vi "EdF.vi"() -> ()   [LabVIEW 2016]
doc: "EdF Test Program - application for testing RadICS platform logic for EdF Project"
uses:
  TypeDef/State.ctl
  TypeDef/Cluster.ctl
  <vilib>/DAQmx/write.llb/DAQmx Write (Digital 1D Bool 1Chan 1Samp).vi
  <vilib>/DAQmx/write.llb/DAQmx Write (Analog 1D DBL NChan 1Samp).vi
  <vilib>/DAQmx/read.llb/DAQmx Read (Digital 1D Bool 1Chan 1Samp).vi
  <vilib>/DAQmx/read.llb/DAQmx Read (Analog 1D DBL NChan 1Samp).vi
  <vilib>/DAQmx/create/channels.llb/DAQmx Create Channel (AO-Voltage-Basic).vi
  <vilib>/DAQmx/create/channels.llb/DAQmx Create Channel (AI-Voltage-Basic).vi
  <vilib>/DAQmx/create/channels.llb/DAQmx Create Channel (DO-Digital Output).vi
  <vilib>/DAQmx/create/channels.llb/DAQmx Create Channel (DI-Digital Input).vi
  <vilib>/DAQmx/miscellaneous.llb/DAQmx Fill In Error Info.vi
  <resource>/objmgr/daqmx.rc
panel:
  in  "PrntScr":bool
  in  "AddTab":enum32{"Page 1"}(tab)
  in  "PID":bool
  in  "Run":bool
  in  "Clear":bool
  out "Graph":dbl[][](graph)
  in  "stop":bool
  in  "Tab":T1(tab)
  in  "AO":tag="6704_S2/ao0:1"
  in  "AI":tag="6224_S4/ai16:21"
  in  "DO":tag="6513_S5/port0/line0:7, 6513_S5/port1/line0:7, 6513_S5/port2/line0"
  in  "DI":tag="6511_S6/port0/line0:7, 6511_S6/port1/line0:3"
  in  "D_out":bool[](array[boolean]) caption="Digital output"
  in  "V_out":dbl[](array[knob]) caption="Analog output,  V" min=0.0 max=5.0 step=1.0 scale=0.0..5.0 scale format="%#.3g"
  in  "AO Names":string[](array[string])=["SRI_2101_MT", "SRI_2203_MT"]
  out "V_in":dbl[](array[numeric]) caption="Analog input, V" format="%.3g"
  in  "AI Names":string[](array[string])=["SRI_01_02_VA_HMI", "SRI_2103_VA_HMI", "SRI_2203MT_HMI", "SRI_2101_VA", "SRI_2102_VA", "SRI_2103_VA"]
  in  "Delay, ms":i32=200
  in  "buf_size":i32=1000 caption="Graph buffer size"
  in  "PID buff":i32=100 caption="PID buffer size"
  in  "DO Names":string[](array[string])=["SRI_2101_RGp_HMI", "SRI_2101_RGm_HMI", "SRI_2101_MA_HMI", "SRI_2150_VN4", "SRI_2160_VN4", "SRI_1201_SN1", "SRI_1202_SN1", "SRI_1203_SN1", "SRI_1201_SN2", "SRI_1202_SN2", "SRI_1203_SN2", "SRI_1101_EE", "SRI_1101_DE", "SRI_1102_EE", "SRI_1102_DE", "SRI_1103_EE", "SRI_1103_DE"]
  out "D_in":bool[](array[boolean]) caption="Digital input"
  in  "DI Names":string[](array[string])=["SRI_2101_AA_HMI", "SRI_2102_AA_HMI", "SRI_1201_AA_HMI", "SRI_1202_AA_HMI", "SRI_1203_AA_HMI", "SER_1201_VA", "SRI_1101_OF", "SRI_1102_OF", "SRI_1103_OF", "SRI_1101_ON", "SRI_1102_ON", "SRI_1103_ON"]
  in  "2203MT":dbl caption="SRI 2203 MT ( C)" min=0.0 max=40.0 step=1.0
  out "03MT":dbl caption="SRI 2203 MT ( C)" format="%.3g"
  out "2103VA":dbl caption="SRI 2103 VA (%)" format="%.3g"
  out "0102VA":dbl caption="SRI 2101/02 VA (%)" format="%.3g"
  in  "2101MT":dbl caption="SRI 2101 MT ( C)" min=0.0 max=40.0 step=1.0
  in  "01RGp":bool caption="SRI 2101 RG+"
  in  "01RGm":bool caption="SRI 2101 RG-"
  in  "01MA":bool caption="SRI 2101 MA"
  in  "50VN4":bool caption="SRI 2150 VN4 (DI)"
  in  "60VN4":bool caption="SRI 2160 VN4 (DI)"
  out "03VA":dbl caption="SRI 2103 VA (%)" format="%.3g"
  out "02AA 2":bool caption="SRI 2102 AA (HMI)"
  out "01AA 2":bool caption="SRI 2101 AA (HMI)"
  out "01VA 2":dbl caption="SRI 2101 VA (%)" format="%.3g"
  out "02VA":dbl caption="SRI 2102 VA (%)" format="%.3g"
  out "03OF":bool caption="SRI 1103 OF (DO)"
  out "01OF":bool caption="SRI 1101 OF (DO)"
  out "02OF":bool caption="SRI 1102 OF (DO)"
  in  "03DE":bool caption="SRI 1103 DE (DI)"
  in  "03EE":bool caption="SRI 1103 EE (DI)"
  in  "02DE":bool caption="SRI 1102 DE (DI)"
  in  "02EE":bool caption="SRI 1102 EE (DI)"
  in  "01DE":bool caption="SRI 1101 DE (DI)"
  out "03ON":bool caption="SRI 1103 ON (DO)"
  out "01ON":bool caption="SRI 1101 ON (DO)"
  out "02ON":bool caption="SRI 1102 ON (DO)"
  in  "01EE":bool caption="SRI 1101 EE (DI)"
  out "03AA":bool caption="SRI 1203 AA"
  out "01VA":bool caption="SER 1201 VA"
  out "02AA":bool caption="SRI 1202 AA"
  in  "01SN1":bool caption="SRI 1201 SN1 (DI)"
  in  "02SN1":bool caption="SRI 1202 SN1 (DI)"
  in  "03SN1":bool caption="SRI 1203 SN1 (DI)"
  in  "01SN2":bool caption="SRI 1201 SN2 (DI)"
  in  "03SN2":bool caption="SRI 1203 SN2 (DI)"
  in  "02SN2":bool caption="SRI 1202 SN2 (DI)"
  out "01AA":bool caption="SRI 1201 AA"
  # "o"
  # "Program Settings"
  # "Closed Loop Control Operation"
  # "0,6648"
  # "0,33"
  # "o"
  # "o"
  # "S0"
  # "D0"
  # "Y"
  # "0,0"
  # "COM"
  # "D1"
  # "0,2"
  # "o"
  # "D0"
  # "Y"
  # "COM"
  # "D1"
  # "S0"
  # "in_1"
  # "out"
  # "OR"
  # "in_2"
  # "op1"
  # "o_result"
  # "SUB"
  # "op2"
  # "op1"
  # "o_result"
  # "MUL"
  # "op2"
  # "op1"
  # "o_result"
  # "MUL"
  # "op2"
  # "o"
  # "17 C"
  # "in_a"
  # "out a<b"
  # "CMP"
  # "in_b"
  # "in_a"
  # "out a>b"
  # "CMP"
  # "in_b"
  # "o"
  # "30 C"
  # "o"
  # "16 C"
  # "op1"
  # "o_result"
  # "SUB"
  # "op2"
  # "i_plus"
  # "o_x_act"
  # "RG"
  # "i_minus"
  # "i_man"
  # "i_x_auto"
  # "o_auto"
  # "i_err"
  # "o_ctrl_val"
  # "PID"
  # "i_prev"
  # "i_auto"
  # "Normal/backup pump operation"
  # "PO3"
  # "PO1"
  # "PO1"
  # "PO2"
  # "PO2"
  # "PO3"
  # "Niv_BAS_01BA"
  # "tctc_vibr"
  # "in"
  # "out"
  # "time: 4000"
  # "in"
  # "out"
  # "NOT"
  # "in"
  # "out"
  # "NOT"
  # "s"
  # "Y"
  # "ff_rs"
  # "r"
  # "tctc_on"
  # "in"
  # "out"
  # "time: 2000"
  # "in_1"
  # "out"
  # "AND"
  # "in_2"
  # "in"
  # "out"
  # "NOT"
  # "in_1"
  # "out"
  # "AND"
  # "in_2"
  # "in_3"
  # "in_1"
  # "out"
  # "OR"
  # "in_2"
  # "in_3"
  # "Alarms"
  # "Niv_BAS_01BA"
  # "in_1"
  # "out"
  # "OR"
  # "in_2"
  # "s"
  # "Y"
  # "ff_rs"
  # "r"
  # "Voter"
  # "in_1"
  # "out"
  # "in_2"
  # "xcount:2"
  # "in_3"
  # "ycount:3"
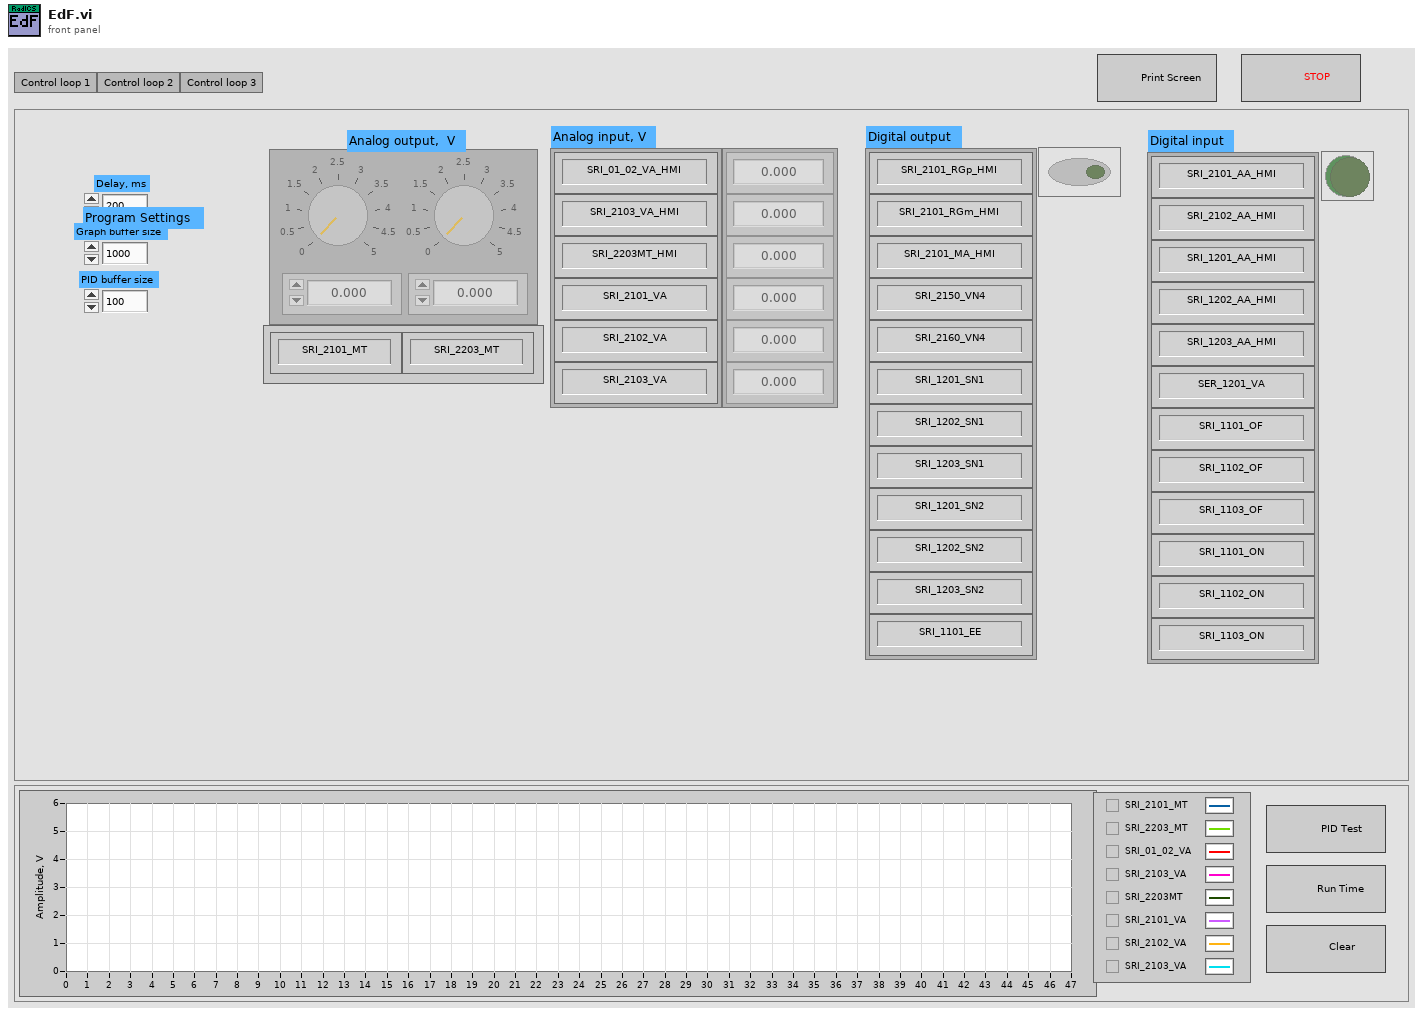
[diagram p1: front panel]
types:
  T1 = enum32{"Manual Control", "Control loop 1", "Control loop 2", "Control loop 3"}
  T2 = typedef "Cluster.ctl" = cluster{"taskAO":refnum<k21>, "taskAI":refnum<k21>, "taskDO":refnum<k21>, "taskDI":refnum<k21>, "UseAO":bool, "UseAI":bool, "UseDO":bool, "UseDI":bool, "Vout":dbl[], "Vin":dbl[], "Dout":bool[], "Din":bool[], "et":dbl, "It":dbl, "Graph":dbl[][], "Index":i32}
  T3 = typedef "State.ctl" = enum16{"Init", "Event", "Alg1", "Alg2", "Alg3", "PID", "Show", "Stop"}
  T4 = cluster{"static gain":dbl, "lag (s)":dbl, "deadtime (s)":dbl, "load":dbl, "deadband":dbl, "sensor noise":dbl, "initial PV":dbl, "plant noise":dbl}
  T5 = typedef "imagedata.ctl" = cluster{"image type":i32, "image depth":i32, "image":u8[], "mask":u8[], "colors":u32[], "Rectangle":cluster{"left":i16, "top":i16, "right":i16, "bottom":i16}}
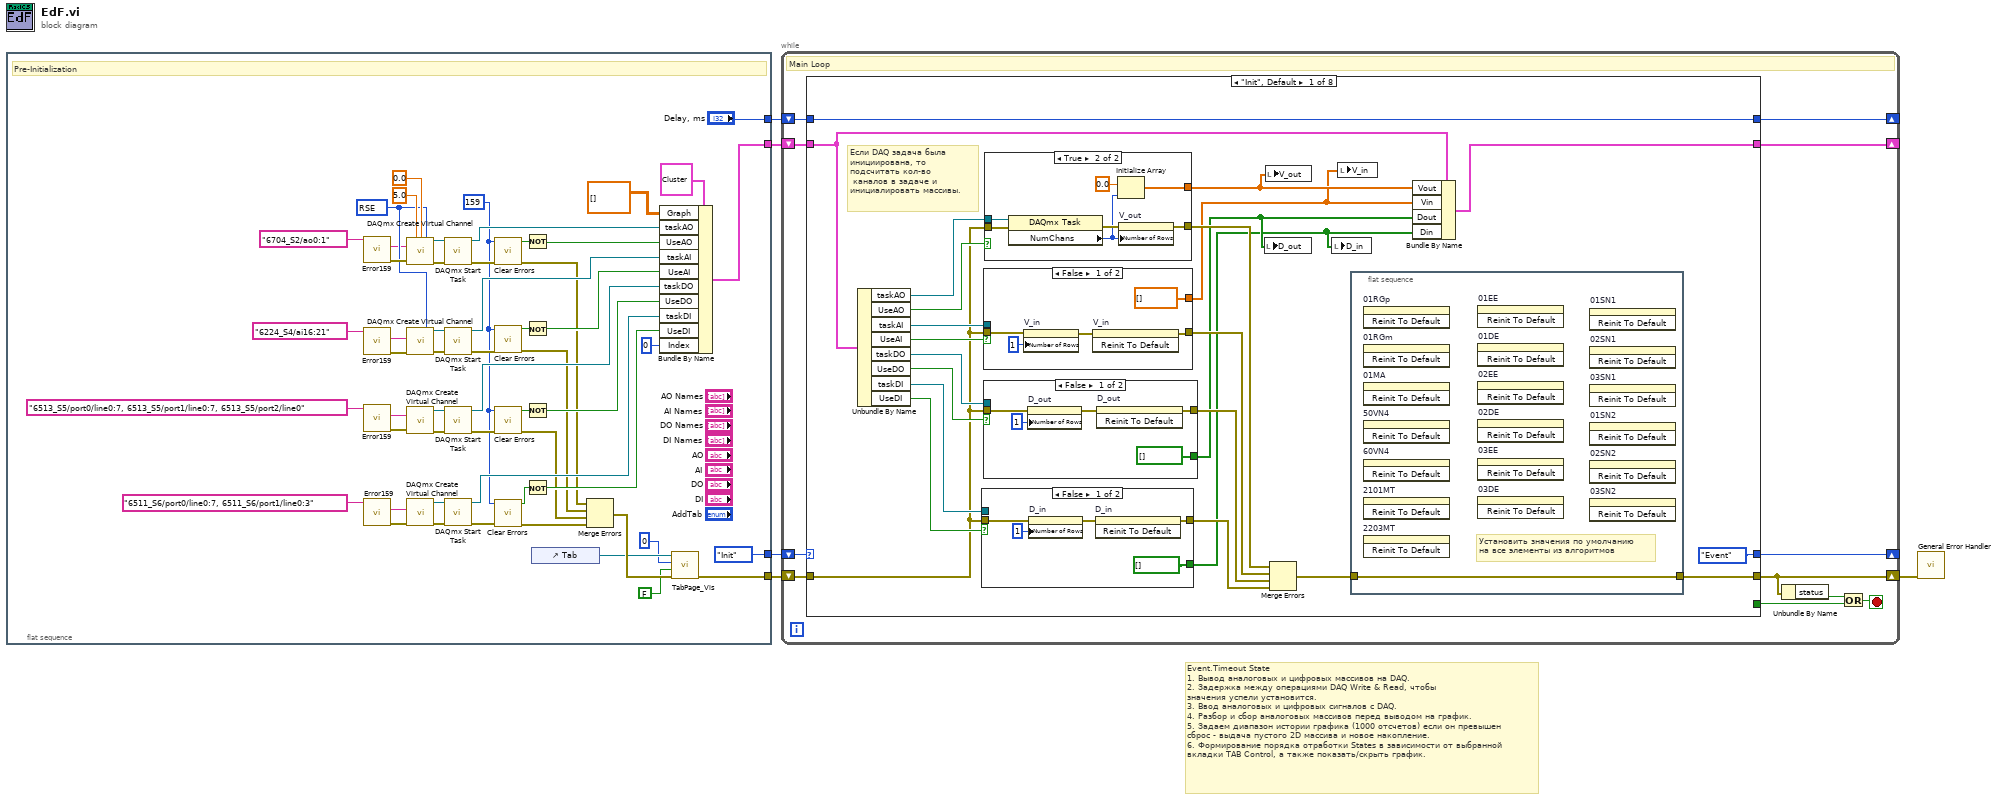
[diagram p0: block diagram]
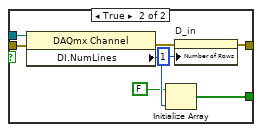
[diagram p2: hidden frame]
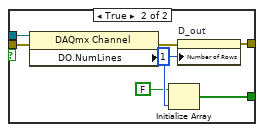
[diagram p3: hidden frame]
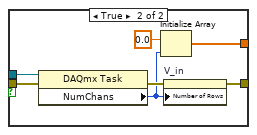
[diagram p4: hidden frame]
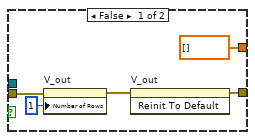
[diagram p5: hidden frame]
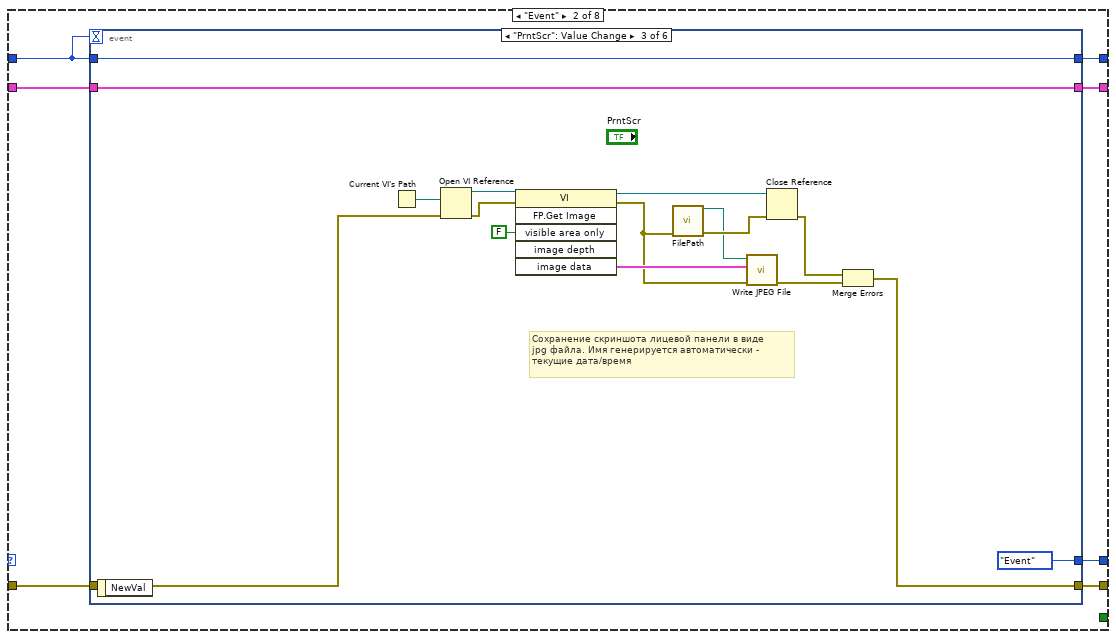
[diagram p6: hidden frame]
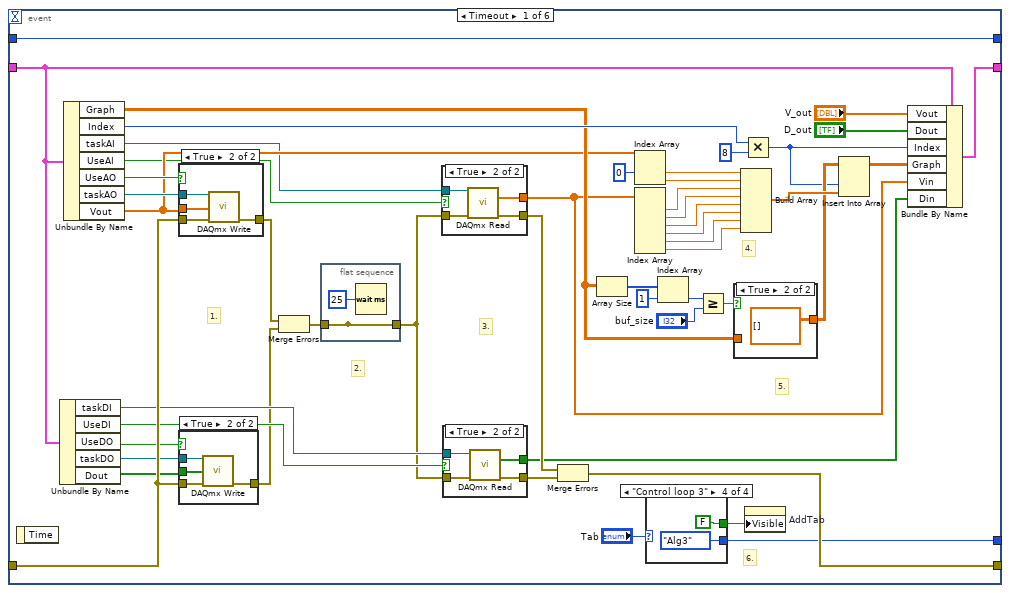
[diagram p7: hidden frame]
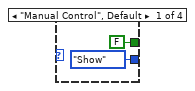
[diagram p8: hidden frame]
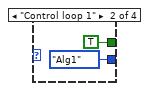
[diagram p9: hidden frame]
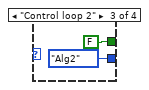
[diagram p10: hidden frame]
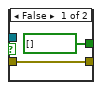
[diagram p12: hidden frame]
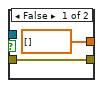
[diagram p14: hidden frame]
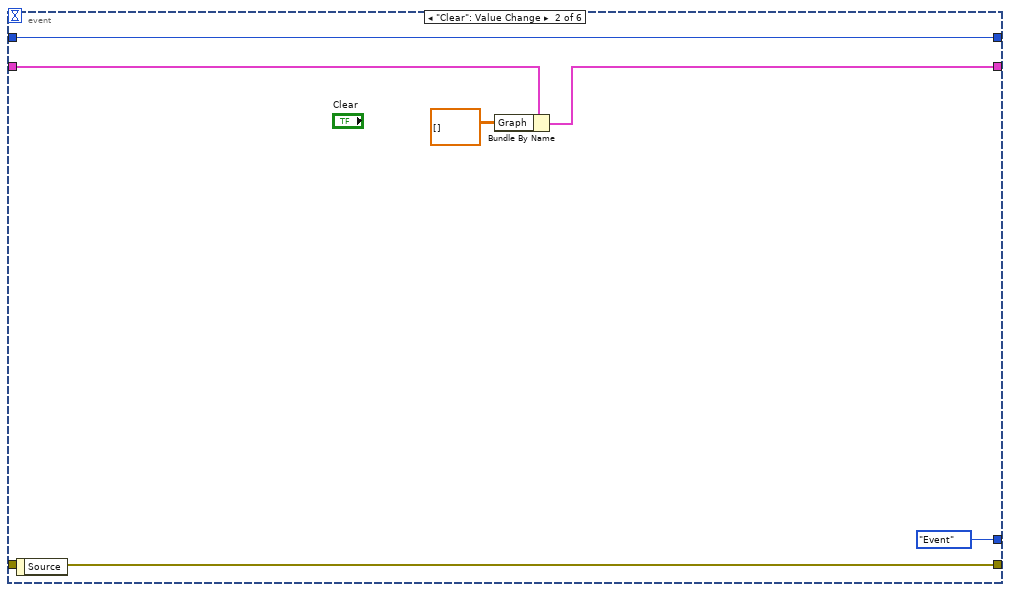
[diagram p16: hidden frame]
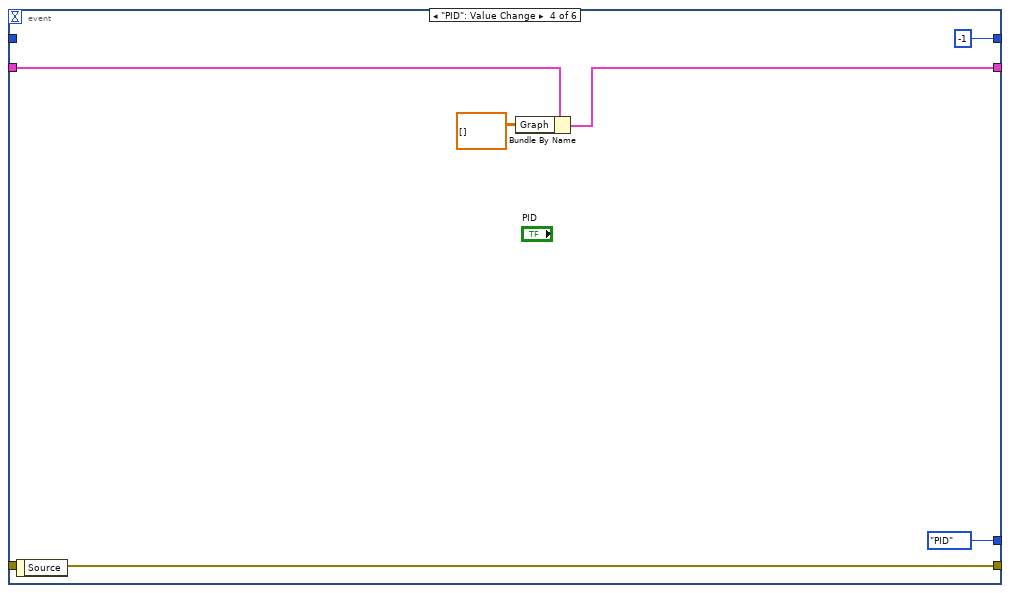
[diagram p17: hidden frame]
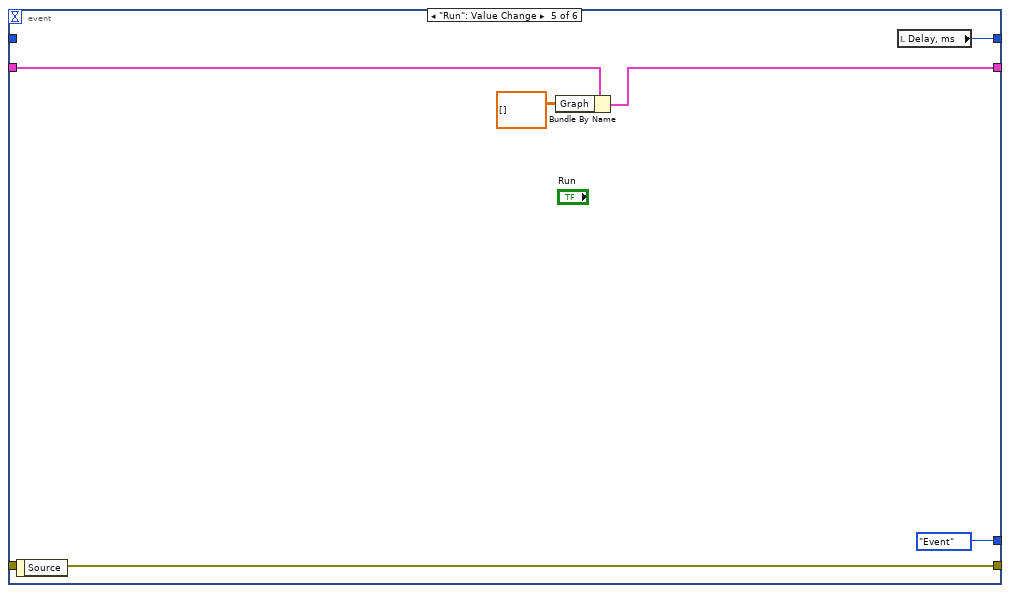
[diagram p18: hidden frame]
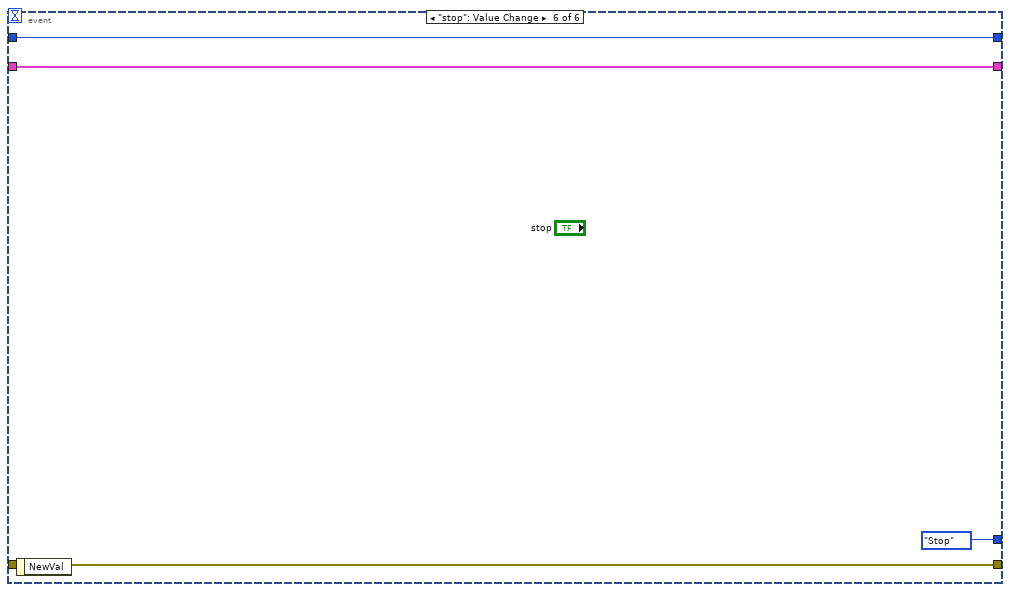
[diagram p19: hidden frame]
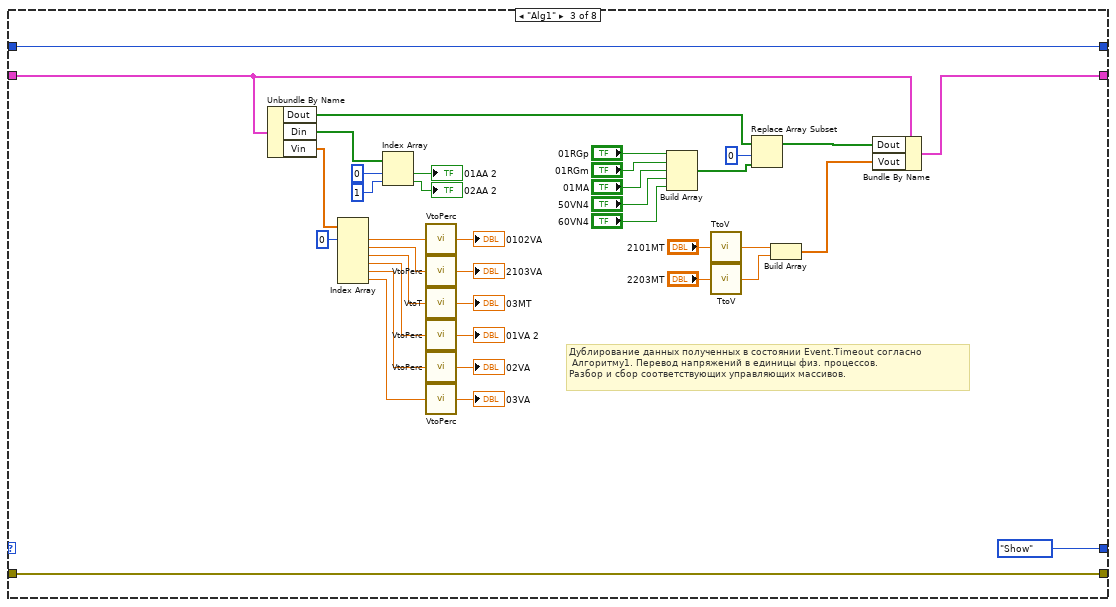
[diagram p20: hidden frame]
diagram:
  # "Event.Timeout State\n1. Вывод аналоговых и цифровых массивов на DAQ.\n2. Задержка между операциями DAQ Write & Read, чтобы\nзначения успели установится.\n3. Ввод аналоговых и цифровых сигналов с DAQ.\n4. Разбор и сбор аналоговых массивов перед выводом на график.\n5. Задаем диапазон истории графика (1000 отсчетов) если он превышен\nсброс - выдача пустого 2D массива и новое накопление.\n6. Формирование порядка отработки States в зависимости от выбранной\nвкладки TAB Control, а также показать/скрыть график."
  n1 = flat-sequence {
    tunnel: [w34] -> w5
    tunnel: ["Delay, ms"] -> w3
    tunnel: [State."Init" ("States")] -> w2
    tunnel: [w10] -> w1
    frame #0 {
      w21 = 10083 items=["Default"=-1, "RSE"=10083, "Differential"=10106, "Pseudodifferential"=12529] ("output terminal configuration")
      w31 = 159 ("specific error code to clear (0: all)")
      # "Pre-Initialization"
      n2 = call "Error159.vi"("Channel"=tag "6704_S2/ao0:1" ("AO")) -> ("error out"=w52:errorcluster, "Channel out"=w20:tag)  [unwired: 9 in]
      n3 = call "Error159.vi"("Channel"=tag "6224_S4/ai16:21" ("AI")) -> ("error out"=w54:errorcluster, "Channel out"=w19:tag)  [unwired: 9 in]
      n4 = call "Error159.vi"("Channel"=tag "6513_S5/port0/line0:7, 6513_S5/port1/line0:7, 6513_S5/port2/line0" ("DO")) -> ("error out"=w53:errorcluster, "Channel out"=w18:tag)  [unwired: 9 in]
      n5 = call "Error159.vi"("Channel"=tag "6511_S6/port0/line0:7, 6511_S6/port1/line0:3" ("DI")) -> ("error out"=w35:errorcluster, "Channel out"=w17:tag)  [unwired: 9 in]
      n6 = call-poly <vilib>:"DAQmx Create Virtual Channel.vi"("maximum value"=5.0, "minimum value"=0.0, "output terminal configuration"=w21, "physical channels"=w20, "error in"=w52) -> ("task out"=w57:refnum<k21>, "error out"=w60:errorcluster)  [unwired: 9 in]
      n7 = call-poly <vilib>:"DAQmx Create Virtual Channel.vi"("input terminal configuration"=w21, "physical channels"=w19, "error in"=w54) -> ("task out"=w56:refnum<k21>, "error out"=w59:errorcluster)  [unwired: 11 in]
      n8 = call-poly <vilib>:"DAQmx Create Virtual Channel.vi"("lines"=w18, "error in"=w53) -> ("task out"=w25:refnum<k21>, "error out"=w24:errorcluster)  [unwired: 12 in]
      n9 = call-poly <vilib>:"DAQmx Create Virtual Channel.vi"("lines"=w17, "error in"=w35) -> ("task out"=w55:refnum<k21>, "error out"=w58:errorcluster)  [unwired: 12 in]
      n10 = call <vilib>:"DAQmx Start Task.vi"("task/channels in"=w57, "error in"=w60) -> ("task out"=w43:refnum<k21>, "error out"=w50:errorcluster)  [unwired: 12 in]
      n11 = call <vilib>:"DAQmx Start Task.vi"("task/channels in"=w56, "error in"=w59) -> ("task out"=w41:refnum<k21>, "error out"=w44:errorcluster)  [unwired: 12 in]
      n12 = call <vilib>:"DAQmx Start Task.vi"("task/channels in"=w25, "error in"=w24) -> ("task out"=w39:refnum<k21>, "error out"=w45:errorcluster)  [unwired: 12 in]
      n13 = call <vilib>:"DAQmx Start Task.vi"("task/channels in"=w55, "error in"=w58) -> ("task out"=w37:refnum<k21>, "error out"=w46:errorcluster)  [unwired: 12 in]
      n14 = call <vilib>:"Clear Errors.vi"("error in (no error)"=w50, "specific error code to clear (0: all)"=w31) -> ("error out"=w29:errorcluster, "specific error cleared?"=w51:bool)  [unwired: 4 in]
      n15 = call <vilib>:"Clear Errors.vi"("error in (no error)"=w44, "specific error code to clear (0: all)"=w31) -> ("error out"=w33:errorcluster, "specific error cleared?"=w49:bool)  [unwired: 4 in]
      n16 = call <vilib>:"Clear Errors.vi"("error in (no error)"=w45, "specific error code to clear (0: all)"=w31) -> ("error out"=w30:errorcluster, "specific error cleared?"=w48:bool)  [unwired: 4 in]
      n17 = call <vilib>:"Clear Errors.vi"("error in (no error)"=w46, "specific error code to clear (0: all)"=w31) -> ("error out"=w32:errorcluster, "specific error cleared?"=w47:bool)  [unwired: 4 in]
      n18 = Not(x=w51) -> (.not. x?=w42:bool)
      n19 = Not(x=w49) -> (.not. x?=w40:bool)
      n20 = Not(x=w48) -> (.not. x?=w38:bool)
      n21 = Not(x=w47) -> (.not. x?=w36:bool)
      n22 = control-ref of="Tab"() -> (w8:refnum<vi>)
      n23 = Merge Errors(w29, w33, w30, w32) -> (w9:errorcluster)
      n24 = Bundle By Name(cluster=T2 {"taskAO"="", "taskAI"="", "taskDO"="", "taskDI"="", "UseAO"=FALSE, "UseAI"=FALSE, "UseDO"=FALSE, "UseDI"=FALSE, "Vout"=[], "Vin"=[], "Dout"=[], "Din"=[], "et"=0.0, "It"=0.0, "Graph"=[], "Index"=0} ("Cluster"), "Graph"=dbl[][] [], "taskAO"=w43, "UseAO"=w42, "taskAI"=w41, "UseAI"=w40, "taskDO"=w39, "UseDO"=w38, "taskDI"=w37, "UseDI"=w36, "Index"=0) -> (w34:T2)
      n25 = call "TabPage_Vis.vi"("error in"=w9, "Visible? (F)"=FALSE ("Visible?"), "Page (0)"=0 ("Page"), "Tab_ref"=w8) -> ("error out"=w10:errorcluster)  [unwired: 7 in]
    }
  }
  n26 = while {
    shift-right: [w62] -> _
    shift-left: w5 -> [w70]
    shift-right: [w69] -> _
    shift-left: w2 -> [w71]
    shift-right: [w67] -> w4
    shift-left: w1 -> [w68]
    shift-right: [w61] -> _
    shift-left: w3 -> [w63]
    stop <- w64 stop-if-true
    # "Main Loop"
    n27 = case shown="\"Init\", Default" w71 {
      tunnel: w70 -> [w81 w152 w294 w328 w350 w361 w439 w464]
      tunnel: [w80 w151 w291 w327 w342 w359 w439 w464] -> w62
      tunnel: [State."Event" ("States") w150 State."Show" ("States") State."Show" ("States") State."Show" ("States") State."Show" ("States") State."Event" ("States") State."Stop" ("States")] -> w69
      tunnel: w68 -> [w86 w149 w309 w334 w354 w365 w441 w457]
      tunnel: [w73 w148 w309 w334 w354 w364 w441 w450] -> w67
      tunnel: [_ _ _ _ _ _ _ TRUE] -> w66
      tunnel: w63 -> [w75 w147 w310 w332 w355 w371 w447 w448]
      tunnel: [w75 w146 w310 w332 w355 w371 w447 w448] -> w61
      frame "Init", Default {
        # "Если DAQ задача была \nинициирована, то\nподсчитать кол-во\n каналов в задаче и \nинициалировать массивы."
        n28 = Unbundle By Name(w81) -> ("taskAO"=w93:refnum<k21>, "UseAO"=w94:bool, "taskAI"=w92:refnum<k21>, "UseAI"=w91:bool, "taskDO"=w90:refnum<k21>, "UseDO"=w89:bool, "taskDI"=w88:refnum<k21>, "UseDI"=w87:bool)
        n29 = case shown="False" w87 {
          tunnel: w88 -> [_ w108]
          tunnel: w86 -> [w100 w104]
          tunnel: [w98 w103] -> w82
          tunnel: [bool[] [] w102] -> w76
          frame False {
            n30 = property on="D_in" class="Arr (strict)"(error in=w100, "Number of Rows"=u32 1 ("Number of Columns")) -> (error out=w99:errorcluster)  [unwired: 1 in, 1 out]
            n31 = invoke on="D_in" class="Arr (strict)" method="Reinit To Default"(error in=w99) -> (error out=w98:errorcluster)  [unwired: 2 in, 2 out]
          }
          frame True {
            n32 = property class="DAQmx Channel"(reference=w108, error in=w104) -> (error out=w107:errorcluster, "DI.NumLines"=w106:u32)  [unwired: 1 out]
            n33 = Initialize Array(FALSE, w106) -> (w102:bool[])
            n34 = property on="D_in" class="Arr (strict)"(error in=w107, "Number of Rows"=u32 1) -> (error out=w103:errorcluster)  [unwired: 1 in, 1 out]
          }
        }
        n35 = case shown="False" w89 {
          tunnel: w90 -> [_ w121]
          tunnel: w86 -> [w111 w117]
          tunnel: [w113 w116] -> w83
          tunnel: [bool[] [] w115] -> w77
          frame False {
            n36 = property on="D_out" class="Arr (strict)"(error in=w111, "Number of Rows"=u32 1 ("Number of Columns")) -> (error out=w112:errorcluster)  [unwired: 1 in, 1 out]
            n37 = invoke on="D_out" class="Arr (strict)" method="Reinit To Default"(error in=w112) -> (error out=w113:errorcluster)  [unwired: 2 in, 2 out]
          }
          frame True {
            n38 = property class="DAQmx Channel"(reference=w121, error in=w117) -> (error out=w120:errorcluster, "DO.NumLines"=w119:u32)  [unwired: 1 out]
            n39 = Initialize Array(FALSE, w119) -> (w115:bool[])
            n40 = property on="D_out" class="Arr (strict)"(error in=w120, "Number of Rows"=u32 1) -> (error out=w116:errorcluster)  [unwired: 1 in, 1 out]
          }
        }
        n41 = case shown="False" w91 {
          tunnel: w92 -> [_ w133]
          tunnel: w86 -> [w126 w129]
          tunnel: [w123 w128] -> w84
          tunnel: [dbl[] [] w127] -> w78
          frame False {
            n42 = property on="V_in" class="Arr (strict)"(error in=w126, "Number of Rows"=u32 1 ("Number of Columns")) -> (error out=w124:errorcluster)  [unwired: 1 in, 1 out]
            n43 = invoke on="V_in" class="Arr (strict)" method="Reinit To Default"(error in=w124) -> (error out=w123:errorcluster)  [unwired: 2 in, 2 out]
          }
          frame True {
            n44 = property class="DAQmx Task"(reference=w133, error in=w129) -> (error out=w132:errorcluster, "NumChans"=w130:u32)  [unwired: 1 out]
            n45 = Initialize Array(0.0 ("element"), w130) -> (w127:dbl[])
            n46 = property on="V_in" class="Arr (strict)"(error in=w132, "Number of Rows"=w130) -> (error out=w128:errorcluster)  [unwired: 1 in, 1 out]
          }
        }
        n47 = case shown="True" w94 {
          tunnel: w93 -> [_ w145]
          tunnel: w86 -> [w138 w139]
          tunnel: [w137 w141] -> w85
          tunnel: [dbl[] [] w140] -> w79
          frame False {
            n48 = property on="V_out" class="Arr (strict)"(error in=w138, "Number of Rows"=u32 1 ("Number of Columns")) -> (error out=w136:errorcluster)  [unwired: 1 in, 1 out]
            n49 = invoke on="V_out" class="Arr (strict)" method="Reinit To Default"(error in=w136) -> (error out=w137:errorcluster)  [unwired: 2 in, 2 out]
          }
          frame True {
            n50 = property class="DAQmx Task"(reference=w145, error in=w139) -> (error out=w144:errorcluster, "NumChans"=w142:u32)  [unwired: 1 out]
            n51 = Initialize Array(0.0 ("element"), w142) -> (w140:dbl[])
            n52 = property on="V_out" class="Arr (strict)"(error in=w144, "Number of Rows"=w142) -> (error out=w141:errorcluster)  [unwired: 1 in, 1 out]
          }
        }
        n53 = local write "D_out"(w77) -> ()
        n54 = local write "V_out"(w79) -> ()
        n55 = Merge Errors(w85, w84, w83, w82) -> (w74:errorcluster)
        n56 = local write "D_in"(w76) -> ()
        n57 = local write "V_in"(w78) -> ()
        n58 = flat-sequence {
          tunnel: w74 -> [w95]
          tunnel: [w95] -> w73
          frame #0 {
            # "Установить значения по умолчанию\nна все элементы из алгоритмов"
            n59 = invoke on="01RGp" class="Bool" method="Reinit To Default"() -> ()  [unwired: 3 in, 3 out]
            n60 = invoke on="01RGm" class="Bool" method="Reinit To Default"() -> ()  [unwired: 3 in, 3 out]
            n61 = invoke on="01MA" class="Bool (strict)" method="Reinit To Default"() -> ()  [unwired: 3 in, 3 out]
            n62 = invoke on="50VN4" class="Bool (strict)" method="Reinit To Default"() -> ()  [unwired: 3 in, 3 out]
            n63 = invoke on="60VN4" class="Bool (strict)" method="Reinit To Default"() -> ()  [unwired: 3 in, 3 out]
            n64 = invoke on="2101MT" class="DigNum (strict)" method="Reinit To Default"() -> ()  [unwired: 3 in, 3 out]
            n65 = invoke on="2203MT" class="DigNum (strict)" method="Reinit To Default"() -> ()  [unwired: 3 in, 3 out]
            n66 = invoke on="01EE" class="Bool (strict)" method="Reinit To Default"() -> ()  [unwired: 3 in, 3 out]
            n67 = invoke on="01DE" class="Bool (strict)" method="Reinit To Default"() -> ()  [unwired: 3 in, 3 out]
            n68 = invoke on="02EE" class="Bool (strict)" method="Reinit To Default"() -> ()  [unwired: 3 in, 3 out]
            n69 = invoke on="02DE" class="Bool (strict)" method="Reinit To Default"() -> ()  [unwired: 3 in, 3 out]
            n70 = invoke on="03EE" class="Bool (strict)" method="Reinit To Default"() -> ()  [unwired: 3 in, 3 out]
            n71 = invoke on="03DE" class="Bool (strict)" method="Reinit To Default"() -> ()  [unwired: 3 in, 3 out]
            n72 = invoke on="01SN1" class="Bool (strict)" method="Reinit To Default"() -> ()  [unwired: 3 in, 3 out]
            n73 = invoke on="02SN1" class="Bool (strict)" method="Reinit To Default"() -> ()  [unwired: 3 in, 3 out]
            n74 = invoke on="03SN1" class="Bool (strict)" method="Reinit To Default"() -> ()  [unwired: 3 in, 3 out]
            n75 = invoke on="01SN2" class="Bool (strict)" method="Reinit To Default"() -> ()  [unwired: 3 in, 3 out]
            n76 = invoke on="02SN2" class="Bool (strict)" method="Reinit To Default"() -> ()  [unwired: 3 in, 3 out]
            n77 = invoke on="03SN2" class="Bool (strict)" method="Reinit To Default"() -> ()  [unwired: 3 in, 3 out]
          }
        }
        n78 = Bundle By Name(cluster=w81, "Vout"=w79, "Vin"=w78, "Dout"=w77, "Din"=w76) -> (w80:T2)
      }
      frame "Event" {
        n79 = event shown="[2] \"PrntScr\": Value Change" {
          selector: _ -> [_ _ _ _ _ _]
          dyn-events: _ -> [_ _ _ _ _ _]
          timeout: w147 -> [_ _ _ _ _ _]
          tunnel: [w196 w237 w257 w259 w264 w273] -> w151
          tunnel: w152 -> [w163 w239 w257 w260 w265 w273]
          tunnel: [w178 State."Event" ("States") State."Event" ("States") State."PID" ("States") State."Event" ("States") State."Stop" ("States")] -> w150
          tunnel: w149 -> [w199 w240 w247 w263 w268 w271]
          tunnel: [w197 w240 w246 w263 w268 w271] -> w148
          tunnel: w147 -> [w181 w236 w242 _ _ w270]
          tunnel: [w181 w236 w242 -1 w267 w270] -> w146
          event Timeout {
            # "6."
            # "5."
            # "4."
            # "3."
            # "2."
            # "1."
            n80 = event-data() -> ()  [unwired: 1 in, 1 out]
            n81 = Unbundle By Name(w163) -> ("taskDI"=w159:refnum<k21>, "UseDI"=w158:bool, "UseDO"=w162:bool, "taskDO"=w161:refnum<k21>, "Dout"=w160:bool[])
            n82 = Unbundle By Name(w163) -> ("Graph"=w185:dbl[][], "Index"=w192:i32, "taskAI"=w165:refnum<k21>, "UseAI"=w164:bool, "UseAO"=w201:bool, "taskAO"=w200:refnum<k21>, "Vout"=w177:dbl[])
            n83 = case shown="True" w201 {
              tunnel: w200 -> [_ w235]
              tunnel: w177 -> [_ w234]
              tunnel: w199 -> [w231 w233]
              tunnel: [w231 w232] -> w157
              frame False {
              }
              frame True {
                n84 = call-poly <vilib>:"DAQmx Write.vi"("task/channels in"=w235, "data"=w234, "error in"=w233) -> ("error out"=w232:errorcluster)  [unwired: 10 in, 2 out]
              }
            }
            n85 = case shown="True" w162 {
              tunnel: w161 -> [_ w222]
              tunnel: w160 -> [_ w221]
              tunnel: w199 -> [w218 w220]
              tunnel: [w218 w219] -> w156
              frame False {
              }
              frame True {
                n86 = call-poly <vilib>:"DAQmx Write.vi"("task/channels in"=w222, "data"=w221, "error in"=w220) -> ("error out"=w219:errorcluster)  [unwired: 10 in, 2 out]
              }
            }
            n87 = Merge Errors(w157, w156) -> (w155:errorcluster)
            n88 = flat-sequence {
              tunnel: w155 -> [w229]
              tunnel: [w229] -> _
              tunnel: [w229] -> w154
              frame #0 {
                n89 = Wait (ms)(milliseconds to wait=u32 25) -> ()  [unwired: 1 out]
              }
            }
            n90 = case shown="True" w164 {
              tunnel: w165 -> [_ w228]
              tunnel: [w223 w227] -> w183
              tunnel: [dbl[] [] ("data") w226] -> w172
              tunnel: w154 -> [w223 w225]
              frame False {
              }
              frame True {
                n91 = call-poly <vilib>:"DAQmx Read.vi"("task/channels in"=w228, "error in"=w225) -> ("data"=w226:dbl[], "error out"=w227:errorcluster)  [unwired: 11 in, 1 out]
              }
            }
            n92 = case shown="True" w158 {
              tunnel: w159 -> [_ w217]
              tunnel: w154 -> [w212 w216]
              tunnel: [w212 w215] -> w198
              tunnel: [bool[] [] ("data") w214] -> w153
              frame False {
              }
              frame True {
                n93 = call-poly <vilib>:"DAQmx Read.vi"("task/channels in"=w217, "error in"=w216) -> ("data"=w214:bool[], "error out"=w215:errorcluster)  [unwired: 11 in, 1 out]
              }
            }
            n94 = Merge Errors(w183, w198) -> (w197:errorcluster)
            n95 = Array Size(array=w185) -> (size(s)=w188:i32[])
            n96 = Index Array(array=w177, index #1=0 ("index")) -> (element #1=w193:dbl, element #2=w173:dbl)  [unwired: 1 in]
            n97 = Index Array(array=w172) -> (element #1=w171:dbl, element #2=w170:dbl, element #3=w169:dbl, element #4=w168:dbl, element #5=w167:dbl, element #6=w166:dbl)  [unwired: 6 in]
            n98 = case shown="\"Control loop 3\"" "Tab" {
              tunnel: [State."Show" ("States") State."Alg1" ("States") State."Alg2" ("States") State."Alg3" ("States")] -> w178
              tunnel: [FALSE TRUE FALSE FALSE] -> w174
              frame "Manual Control", Default {
              }
              frame "Control loop 1" {
              }
              frame "Control loop 2" {
              }
              frame "Control loop 3" {
              }
            }
            n99 = Index Array(array=w188, index=1) -> (element=w186:i32)
            n100 = Greater Or Equal?(x=w186, y="buf_size") -> (x >= y?=w190:bool)
            n101 = case shown="True" w190 {
              tunnel: w185 -> [w210 _]
              tunnel: [w210 dbl[][] []] -> w184
              frame False {
              }
              frame True {
              }
            }
            n102 = Build Array(w193, w173, w171, w170, w169, w168, w167, w166) -> (w191:dbl[])
            n103 = Multiply(x=w192, y=8) -> (x*y=w180:i32)
            n104 = property on="AddTab" class="TabCtl (strict)"("Visible"=w174) -> ()  [unwired: 2 in, 2 out]
            n105 = Insert Into Array(array=w184, index (col)=w180, new element=w191) -> (w195:dbl[][])  [unwired: 1 in]
            n106 = Bundle By Name(cluster=w163, "Vout"="V_out", "Dout"="D_out", "Index"=w180, "Graph"=w195, "Vin"=w172, "Din"=w153) -> (w196:T2)
          }
          event "Clear": Value Change {
            n107 = event-data() -> ()  [unwired: 1 in, 1 out]
            n108 = Bundle By Name(cluster=w239, "Graph"=dbl[][] []) -> (w237:T2)
          }
          event "PrntScr": Value Change {
            # "Сохранение скриншота лицевой панели в виде\njpg файла. Имя генерируется автоматически - \nтекущие дата/время"
            n109 = event-data() -> ()  [unwired: 1 in, 1 out]
            n110 = Current VI's Path() -> (path=w248:path)
            n111 = Open VI Reference(vi path=w248, error in (no error)=w247) -> (vi reference=w255:refnum<vi>, error out=w254:errorcluster)  [unwired: 4 in]
            n112 = invoke class="VI" method="FP.Get Image"(reference=w255, error in=w254, "visible area only"=FALSE ("Visible Area Only")) -> (reference out=w253:refnum<vi>, error out=w243:errorcluster, "image data"=w252:T5)  [unwired: 3 in, 3 out]
            n113 = call "FilePath.vi"("error in"=w243) -> ("error out"=w245:errorcluster, "File path"=w244:path)  [unwired: 9 in]
            n114 = call <vilib>:"Write JPEG File.vi"("error in (no error)"=w243, "image data"=w252, "path to JPEG file"=w244) -> ("error out"=w251:errorcluster)  [unwired: 7 in, 1 out]
            n115 = Close Reference(reference=w253, error in (no error)=w245) -> (error out=w250:errorcluster)
            n116 = Merge Errors(w250, w251) -> (w246:errorcluster)
          }
          event "PID": Value Change {
            n117 = event-data() -> ()  [unwired: 1 in, 1 out]
            n118 = Bundle By Name(cluster=w260, "Graph"=dbl[][] []) -> (w259:T2)
          }
          event "Run": Value Change {
            n119 = event-data() -> ()  [unwired: 1 in, 1 out]
            n120 = Bundle By Name(cluster=w265, "Graph"=dbl[][] []) -> (w264:T2)
            n121 = local read "Delay, ms"() -> (w267:i32)
          }
          event "stop": Value Change {
            n122 = event-data() -> ()  [unwired: 1 in, 1 out]
          }
        }
      }
      frame "Alg1" {
        # "Дублирование данных полученных в состоянии Event.Timeout согласно\n Алгоритму1. Перевод напряжений в единицы физ. процессов.\nРазбор и сбор соответствующих управляющих массивов."
        n123 = Unbundle By Name(w294) -> ("Dout"=w296:bool[], "Din"=w306:bool[], "Vin"=w295:dbl[])
        n124 = Index Array(array=w295, index #1=0 ("index")) -> (element #1=w286:dbl, element #2=w285:dbl, element #3=w284:dbl, element #4=w283:dbl, element #5=w282:dbl, element #6=w281:dbl)  [unwired: 5 in]
        n125 = Index Array(array=w306, index #1=0 ("index"), index #2=1 ("index")) -> (element #1=→"01AA 2":bool, element #2=→"02AA 2":bool)
        n126 = call "VtoPerc.vi"("Volt"=w286) -> ("Perc"=→"0102VA":dbl)
        n127 = call "VtoPerc.vi"("Volt"=w285) -> ("Perc"=→"2103VA":dbl)
        n128 = call "VtoT.vi"("Volt"=w284) -> ("Temp"=→"03MT":dbl)
        n129 = call "VtoPerc.vi"("Volt"=w283) -> ("Perc"=→"01VA 2":dbl)
        n130 = call "VtoPerc.vi"("Volt"=w282) -> ("Perc"=→"02VA":dbl)
        n131 = call "VtoPerc.vi"("Volt"=w281) -> ("Perc"=→"03VA":dbl)
        n132 = Build Array("01RGp", "01RGm", "01MA", "50VN4", "60VN4") -> (w307:bool[])
        n133 = call "TtoV.vi"("Temp"="2101MT") -> ("Volt"=w290:dbl)
        n134 = call "TtoV.vi"("Temp"="2203MT") -> ("Volt"=w289:dbl)
        n135 = Replace Array Subset(array=w296, new element=w307, index=0) -> (w293:bool[])
        n136 = Build Array(w290, w289) -> (w292:dbl[])
        n137 = Bundle By Name(cluster=w294, "Dout"=w293, "Vout"=w292) -> (w291:T2)
      }
      frame "Alg2" {
        # "Дублирование данных полученных в состоянии\n Event.Timeout согласно Алгоритму2. Разбор и \nсбор соответствующих управляющих массивов"
        n138 = Unbundle By Name(w328) -> ("Dout"=w329:bool[], "Din"=w325:bool[])
        n139 = Index Array(array=w325, index #1=6 ("index")) -> (element #1=→"01OF":bool, element #2=→"02OF":bool, element #3=→"03OF":bool, element #4=→"01ON":bool, element #5=→"02ON":bool, element #6=→"03ON":bool)  [unwired: 5 in]
        n140 = Build Array("01EE", "01DE", "02EE", "02DE", "03EE", "03DE") -> (w326:bool[])
        n141 = Replace Array Subset(array=w329, new element=w326, index=11) -> (w317:bool[])
        n142 = Bundle By Name(cluster=w328, "Dout"=w317) -> (w327:T2)
      }
      frame "Alg3" {
        # "Дублирование данных полученных в состоянии\n Event.Timeout согласно Алгоритму3. Разбор и \nсбор соответствующих управляющих массивов"
        n143 = Unbundle By Name(w350) -> ("Dout"=w343:bool[], "Din"=w339:bool[])
        n144 = Index Array(array=w339, index #1=2 ("index")) -> (element #1=→"01AA":bool, element #2=→"02AA":bool, element #3=→"03AA":bool, element #4=→"01VA":bool)  [unwired: 3 in]
        n145 = Build Array("01SN1", "02SN1", "03SN1", "01SN2", "02SN2", "03SN2") -> (w344:bool[])
        n146 = Replace Array Subset(array=w343, new element=w344, index=5) -> (w338:bool[])
        n147 = Bundle By Name(cluster=w350, "Dout"=w338) -> (w342:T2)
      }
      frame "PID" {
        # "Реализация двух подходов для проверки ПИД регулятора.\nЧтение запись с DAQ происходит в цыкле, поэтому на графике\nданные отобразятся после полной его отработки указанное\nчисло итераций (100)"
        n148 = Unbundle By Name(w361) -> ("Graph"=w363:dbl[][], "taskAO"=w367:refnum<k21>, "taskAI"=w366:refnum<k21>, "UseAO"=w370:bool, "UseAI"=w369:bool, "Vout"=w357:dbl[])
        n149 = And(x=w370, y=w369) -> (x .and. y?=w368:bool)
        n150 = case shown="True" w368 {
          tunnel: w367 -> [_ w382]
          tunnel: w366 -> [_ w381]
          tunnel: w365 -> [w374 w380]
          tunnel: [w374 w379] -> w364
          tunnel: [dbl[][] [] w378] -> w356
          tunnel: w357 -> [_ w376]
          frame False {
            # "Если хоть один из модулей не инициирован\nничего не выполнять, на график 0"
          }
          frame True {
            n151 = case shown="\"Model\"" enum16{"OldPID", "Model"}."OldPID" {
              tunnel: w382 -> [w389 w416]
              tunnel: w381 -> [w388 w415]
              tunnel: w380 -> [w387 w414]
              tunnel: [w386 w413] -> w379
              tunnel: [w385 w412] -> w378
              tunnel: "PID buff" -> [w384 w410]
              tunnel: w376 -> [w383 w409]
              frame "Model" {
                n152 = for {
                  N: w384 -> [_]
                  tunnel: w389 -> [w403]
                  tunnel: w388 -> [w405]
                  shift-right: [w400] -> w386
                  shift-left: w387 -> [w404]
                  tunnel: [w406] -> w385 mode=indexing
                  tunnel: w383 -> [w402]
                  # "формир соотв. кол-во эл-в в массиве для графика"
                  n153 = call-poly <vilib>:"DAQmx Read.vi"("task/channels in"=w405, "error in"=w404) -> ("data"=w396:dbl[], "error out"=w390:errorcluster)  [unwired: 11 in, 1 out]
                  n154 = Index Array(array=w396, index=0) -> (element=w392:dbl)
                  n155 = call "Plant System.vi"("output saturation range"=cluster{"output high":dbl, "output low":dbl} {"output high"=5.0, "output low"=0.0}, "Plant Input"=w392, "process parameters"=T4 {"static gain"=1.0, "lag (s)"=1.0, "deadtime (s)"=0.001, "load"=0.0, "deadband"=0.0, "sensor noise"=0.0, "initial PV"=0.5, "plant noise"=0.0}) -> ("Plant Output"=w391:dbl)  [unwired: 12 in]
                  n156 = flat-sequence {
                    tunnel: w390 -> [w408]
                    tunnel: [w408] -> w401
                    frame #0 {
                      n157 = Wait (ms)(milliseconds to wait=u32 25) -> ()  [unwired: 1 out]
                    }
                  }
                  n158 = Replace Array Subset(array=w402, new element=w391, index=0) -> (w395:dbl[])
                  n159 = Insert Into Array(array=w396, index=0, new element=w395) -> (w406:dbl[])
                  n160 = call-poly <vilib>:"DAQmx Write.vi"("task/channels in"=w403, "data"=w395, "error in"=w401) -> ("error out"=w400:errorcluster)  [unwired: 10 in, 2 out]
                }
              }
              frame "OldPID", Default {
                n161 = for {
                  N: w410 -> [_]
                  tunnel: w416 -> [w430]
                  tunnel: w415 -> [w435]
                  shift-right: [w424] -> w413
                  shift-left: w414 -> [w434]
                  tunnel: [w436] -> w412 mode=indexing
                  tunnel: w409 -> [w429]
                  shift-right: [w425] -> _
                  shift-left: 0.0 ("element") -> [w426]
                  # "формир соотв. кол-во эл-в в массиве для графика"
                  n162 = call-poly <vilib>:"DAQmx Read.vi"("task/channels in"=w435, "error in"=w434) -> ("data"=w418:dbl[], "error out"=w433:errorcluster)  [unwired: 11 in, 1 out]
                  n163 = Index Array(array=w418, index=0) -> (element=w423:dbl)
                  n164 = call "PID_old.vi"("(t-1)in"=w426, "error in"=w433, "Low_Limit (0)"=13.0 ("Low_Limit"), "Up_Limit (40)"=40.0 ("Up_Limit"), "Ain"=w423) -> ("error out"=w428:errorcluster, "Aout"=w419:dbl, "(t-1)out"=w425:dbl)  [unwired: 4 in]
                  n165 = flat-sequence {
                    tunnel: w428 -> [w438]
                    tunnel: [w438] -> w427
                    frame #0 {
                      n166 = Wait (ms)(milliseconds to wait=u32 25) -> ()  [unwired: 1 out]
                    }
                  }
                  n167 = Replace Array Subset(array=w429, new element=w419, index=0) -> (w417:dbl[])
                  n168 = Insert Into Array(array=w418, index=0, new element=w417) -> (w436:dbl[])
                  n169 = call-poly <vilib>:"DAQmx Write.vi"("task/channels in"=w430, "data"=w417, "error in"=w427) -> ("error out"=w424:errorcluster)  [unwired: 10 in, 2 out]
                }
              }
            }
          }
        }
        n170 = Transpose 2D Array(2D array=w356) -> (transposed array=w358:dbl[][])
        n171 = Insert Into Array(array=w363, index (col)=0 ("disabled index (col)"), new element=w358) -> (w360:dbl[][])  [unwired: 1 in]
        n172 = Bundle By Name(cluster=w361, "Graph"=w360) -> (w359:T2)
      }
      frame "Show" {
        n173 = Unbundle By Name(w439) -> ("Graph"=→"Graph":dbl[][], "Dout"=w443:bool[], "Din"=→"D_in":bool[], "Vin"=→"V_in":dbl[], "Vout"=w446:dbl[])
        n174 = local write "D_out"(w443) -> ()
        n175 = local write "V_out"(w446) -> ()
      }
      frame "Stop" {
        # "Если DAQ задача была инициирована\n- остановить и очистить ее"
        n176 = Unbundle By Name(w464) -> ("taskAO"=w462:refnum<k21>, "UseAO"=w463:bool, "taskAI"=w460:refnum<k21>, "UseAI"=w461:bool, "taskDO"=w458:refnum<k21>, "UseDO"=w459:bool, "taskDI"=w456:refnum<k21>, "UseDI"=w455:bool)
        n177 = case shown="True" w463 {
          tunnel: w462 -> [_ w488]
          tunnel: w457 -> [w484 w486]
          tunnel: [w484 w485] -> w454
          frame False {
          }
          frame True {
            n178 = call <vilib>:"DAQmx Stop Task.vi"("task/channels in"=w488, "error in"=w486) -> ("task out"=w487:refnum<k21>, "error out"=w489:errorcluster)  [unwired: 12 in]
            n179 = call <vilib>:"DAQmx Clear Task.vi"("task in"=w487, "error in"=w489) -> ("error out"=w485:errorcluster)  [unwired: 13 in]
          }
        }
        n180 = case shown="True" w461 {
          tunnel: w457 -> [w478 w482]
          tunnel: [w478 w481] -> w453
          tunnel: w460 -> [_ w480]
          frame False {
          }
          frame True {
            n181 = call <vilib>:"DAQmx Stop Task.vi"("task/channels in"=w480, "error in"=w482) -> ("task out"=w479:refnum<k21>, "error out"=w483:errorcluster)  [unwired: 12 in]
            n182 = call <vilib>:"DAQmx Clear Task.vi"("task in"=w479, "error in"=w483) -> ("error out"=w481:errorcluster)  [unwired: 13 in]
          }
        }
        n183 = case shown="True" w459 {
          tunnel: w457 -> [w472 w476]
          tunnel: [w472 w475] -> w452
          tunnel: w458 -> [_ w473]
          frame False {
          }
          frame True {
            n184 = call <vilib>:"DAQmx Stop Task.vi"("task/channels in"=w473, "error in"=w476) -> ("task out"=w474:refnum<k21>, "error out"=w477:errorcluster)  [unwired: 12 in]
            n185 = call <vilib>:"DAQmx Clear Task.vi"("task in"=w474, "error in"=w477) -> ("error out"=w475:errorcluster)  [unwired: 13 in]
          }
        }
        n186 = case shown="True" w455 {
          tunnel: w457 -> [w466 w467]
          tunnel: w456 -> [_ w470]
          tunnel: [w466 w469] -> w451
          frame False {
          }
          frame True {
            n187 = call <vilib>:"DAQmx Stop Task.vi"("task/channels in"=w470, "error in"=w467) -> ("task out"=w468:refnum<k21>, "error out"=w471:errorcluster)  [unwired: 12 in]
            n188 = call <vilib>:"DAQmx Clear Task.vi"("task in"=w468, "error in"=w471) -> ("error out"=w469:errorcluster)  [unwired: 13 in]
          }
        }
        n189 = Merge Errors(w454, w453, w452, w451) -> (w450:errorcluster)
      }
    }
    n190 = Unbundle By Name(w67) -> ("status"=w65:bool)
    n191 = Or(x=w65, y=w66) -> (x .or. y?=w64:bool)
  }
  n192 = call <vilib>:"General Error Handler.vi"("error in (no error)"=w4) -> ()  [unwired: 10 in, 5 out]
